vi "E11_GraficoIntensidad.vi"() -> ()   [LabVIEW 2026]
panel:
  in  "Columnas":i32
  in  "Filas":i32
  out "Intensity Graph":dbl[][](graph)
  out "Array":dbl[][](array[numeric])
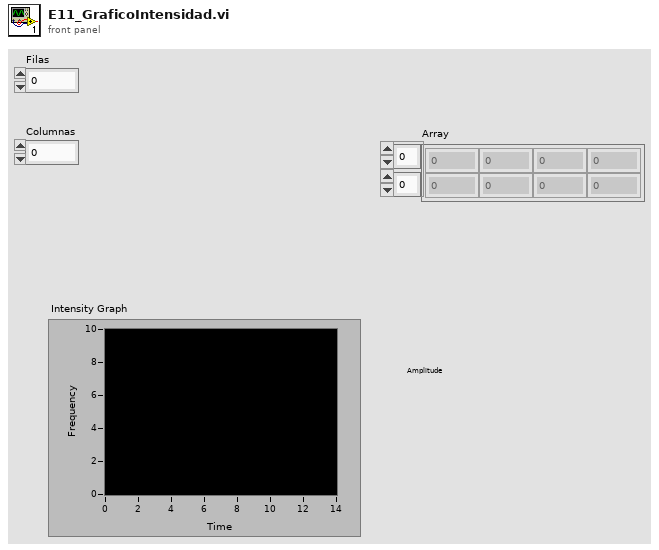
[diagram p1: front panel]
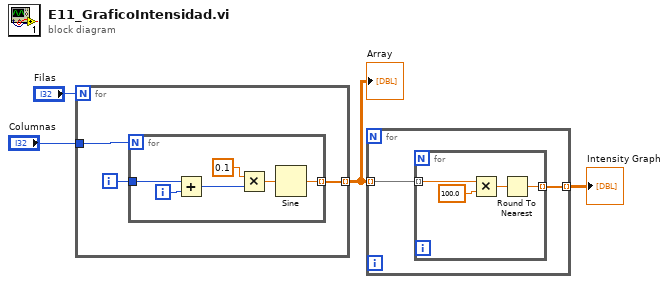
[diagram p0: block diagram]
diagram:
  n1 = for {
    N: "Filas" -> [_]
    tunnel: [w6] -> w1 mode=indexing
    tunnel: "Columnas" -> [w5]
    i -> [w7]
    n2 = for {
      N: w5 -> [_]
      tunnel: w7 -> [w11]
      tunnel: [w8] -> w6 mode=indexing
      i -> [w12]
      n3 = Add(x=w11, y=w12) -> (x+y=w10:i32)
      n4 = Multiply(x=0.1, y=w10) -> (x*y=w13:dbl)
      n5 = Sine(x=w13) -> (sin(x)=w8:dbl)
    }
  }
  "Array" <- w1
  n6 = for {
    tunnel: [w15] -> w4 mode=indexing
    tunnel: w1 -> [w14] mode=indexing
    n7 = for {
      tunnel: [w18] -> w15 mode=indexing
      tunnel: w14 -> [w16] mode=indexing
      n8 = Multiply(x=w16, y=100.0) -> (x*y=w19:dbl)
      n9 = Round To Nearest(number=w19) -> (nearest integer value=w18:dbl)
    }
  }
  "Intensity Graph" <- w4
